vi "Write Single ELAN Value.vi"(8 "error in (no error)":errorcluster, 9 "Value":T1 {"Value"."Value" format="%#_6f"}, 10 "address":u16, 11 "device data model in":refnum<class "Device Data Model.lvclass">) -> (0 "error out":errorcluster, 3 "device data model out":refnum<class "Device Data Model.lvclass">)   [LabVIEW 2021, in "Device Data Model.lvclass"]
doc: "Writes the value of a single holding register."
uses:
  Device Data Model.lvclass
  Master CR/Data Model/ELAN Data Model/Type Definitions/Value full.ctl
  Master CR/Data Unit/ELAN PC Data Unit/Elan units.ctl
  Master CR/Data Unit/ELAN PC Data Unit/Elan measured variable.ctl
  Master CR/Data Unit/ELAN PC Data Unit/Elan channel state.ctl
  Master CR/Data Unit/ELAN PC Data Unit/ELAN PDU.lvclass
  Master CR/Data Model/ELAN Data Model/ELAN Data Model.lvclass
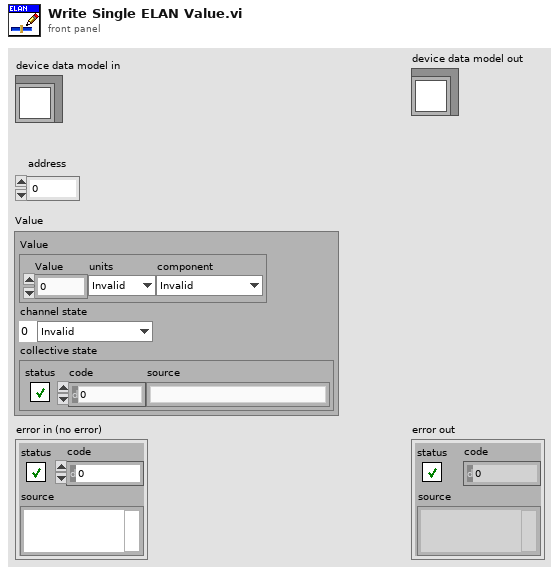
[diagram p1: front panel]
types:
  T1 = typedef "ELAN Data Model.lvclass/Value full.ctl" = cluster{"Value":cluster{"Value":sgl, "units":T2, "component":T3}, "channel state":T4, "collective state":errorcluster}
  T2 = typedef "ELAN PDU.lvclass/Elan units.ctl" = enum16{"Invalid", "no dimension", "ppm", "ppb", "vpm", "ppm C1", "ppm C3", "ppm C6", "mg C/m3", "mg/m3", "%", "% vol", "% of measuring range", "% saturation", "%/°C", "%/K", "% weight", "mV/pH", "mV/mbar", "nA/mbar", "S/m", "S/cm", "mS/m", "mS/cm", "ìS/m", "ìS/cm", "S", "min", "H", "Pa", "MA", "uV", "MV", "V", "mbar", "hPa", "Ml/min", "kOhm", "MOhm", "S1", "°C", "Hz", "pH", "ug/l", "mg/l", "l/min", "uA", "mg/dm3", "kPa", "kOhm*cm", "MOhm*cm", "°", "1/min", "1/m", "g/m3", "g/l", "% Vol C"}
  T3 = typedef "ELAN PDU.lvclass/Elan measured variable.ctl" = enum16{"Invalid", "no component", "CO", "CO2", "CH4 (Methan)", "C6H14 (Hexan)", "SO2", "NO", "NO2", "CHClF2 (R22)", "C3H8 (Propan)", "C4H10 (Butan)", "O2", "C5H12 (Pentan)", "CnHm (THC)", "P (process pressure)", "pH", "T (temperature)", "C2H4 (Ethen)", "C2H2 (Ethin)", "C3H6 (Propen)", "C4H6", "C4H8", "C2H6", "NH3 (Ammoniak)", "N2O", "C6H6 (Benzol)", "SF6", "CH3OH (Methanol)", "C2H5OH (Ethanol)", "CH2Cl2", "C2H4Cl2", "CH3Cl", "C2H4O", "H2O (water vapor)", "G/l (conductivity)", "C", "S", "N", "CF4", "COCl2 (phosgene)", "CHF3 (R23)", "C2F6 (R116)", "------ (self defined component)", "C2H3Cl", "H2 (Hydrogen)", "Ar", "He", "Cl2", "N2"}
  T4 = typedef "ELAN PDU.lvclass/Elan channel state.ctl" = enum16{"Invalid", "Warm-up", "Pause", "Standby", "Measure", "Zero calibration", "Adjust component slope", "Not yet defined1", "Adjust curve dip", "Adjust linearization sensitivity", "Adjust temperature compensation", "Adjust pressure compensation", "Adjust linearization zero", "Not yet defined2", "Autocal", "Adjust phase", "Zero calibration of O2 sensor", "Synchronous zero calibration", "Purging for synchronous zero calibration", "Adjust analog output", "Adjust analog input", "Autocal check"}
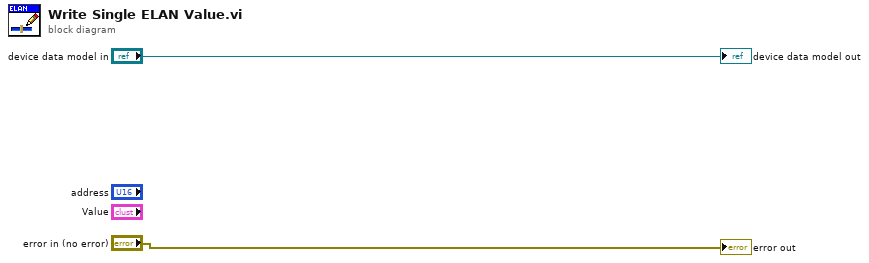
[diagram p0: block diagram]
diagram:
  "error out" <- "error in (no error)"
  "device data model out" <- "device data model in"
